vi "Latihan 8 (Case Structure).vi"() -> ()   [LabVIEW 2021]
panel:
  out "Hasil":dbl
  in  "Angka Kedua":dbl
  in  "Angka Pertama":dbl
  in  "Opsi":enum16{"Kali", "Bagi", "Kurang", "Tambah"}(ring)
  in  "\"=\"":bool
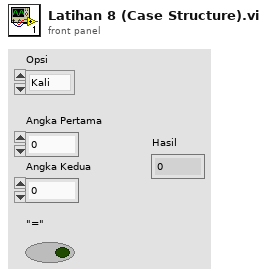
[diagram p1: front panel]
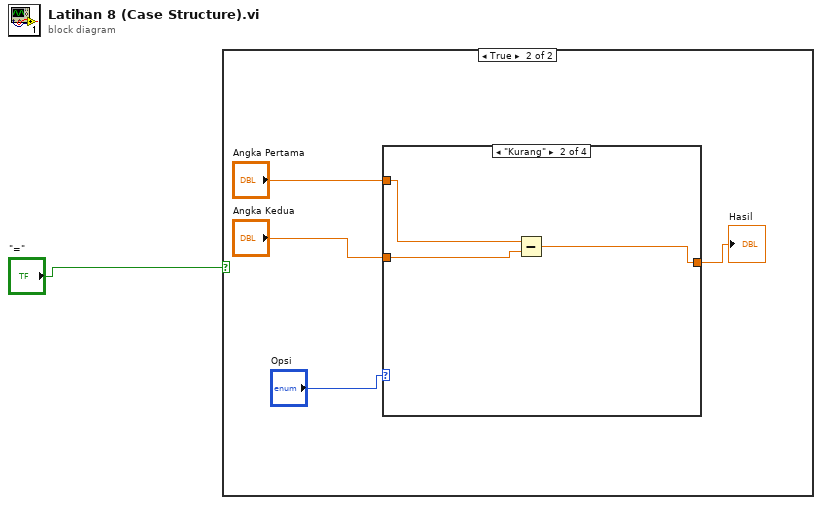
[diagram p0: block diagram]
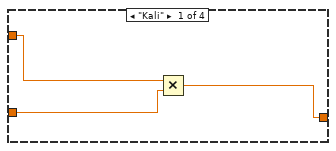
[diagram p3: hidden frame]
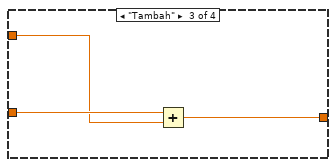
[diagram p4: hidden frame]
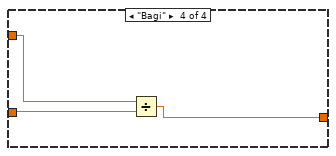
[diagram p5: hidden frame]
diagram:
  n1 = case shown="True" "\"=\"" {
    frame False {
    }
    frame True {
      n2 = case shown="\"Kurang\"" "Opsi" {
        tunnel: "Angka Kedua" -> [w7 w10 w14 w16]
        tunnel: "Angka Pertama" -> [w8 w11 w13 w17]
        tunnel: [w6 w9 w12 w15] -> w2
        frame "Kali" {
          n3 = Multiply(x=w8, y=w7) -> (x*y=w6:dbl)
        }
        frame "Kurang" {
          n4 = Subtract(x=w11, y=w10) -> (x-y=w9:dbl)
        }
        frame "Tambah" {
          n5 = Add(x=w14, y=w13) -> (x+y=w12:dbl)
        }
        frame "Bagi" {
          n6 = Divide(x=w17, y=w16) -> (x/y=w15:dbl)
        }
      }
      "Hasil" <- w2
    }
  }
